vi "Cam1.vi"(1 "error in (no error)":errorcluster) -> (0 "error out":errorcluster caption="error in (no error)")   [LabVIEW 2018]
uses:
  InOut/Reslut.vi
  VsyCam.dll
panel:
  out "当前曝光":dbl
  out "近场图":T1(plugin-control)
  in  "重新连接相机":bool
  out "帧率":dbl
  in  "采集":bool
  in  "数据输出":i32[](listbox)
  out "通信":bool
  out "远场图":T1(plugin-control)
  in  "触发方式":enum8{"软件触发", "上升沿触发", "下降沿触发"}(ring)
  in  "曝光设置 us":i32 min=1 max=2000
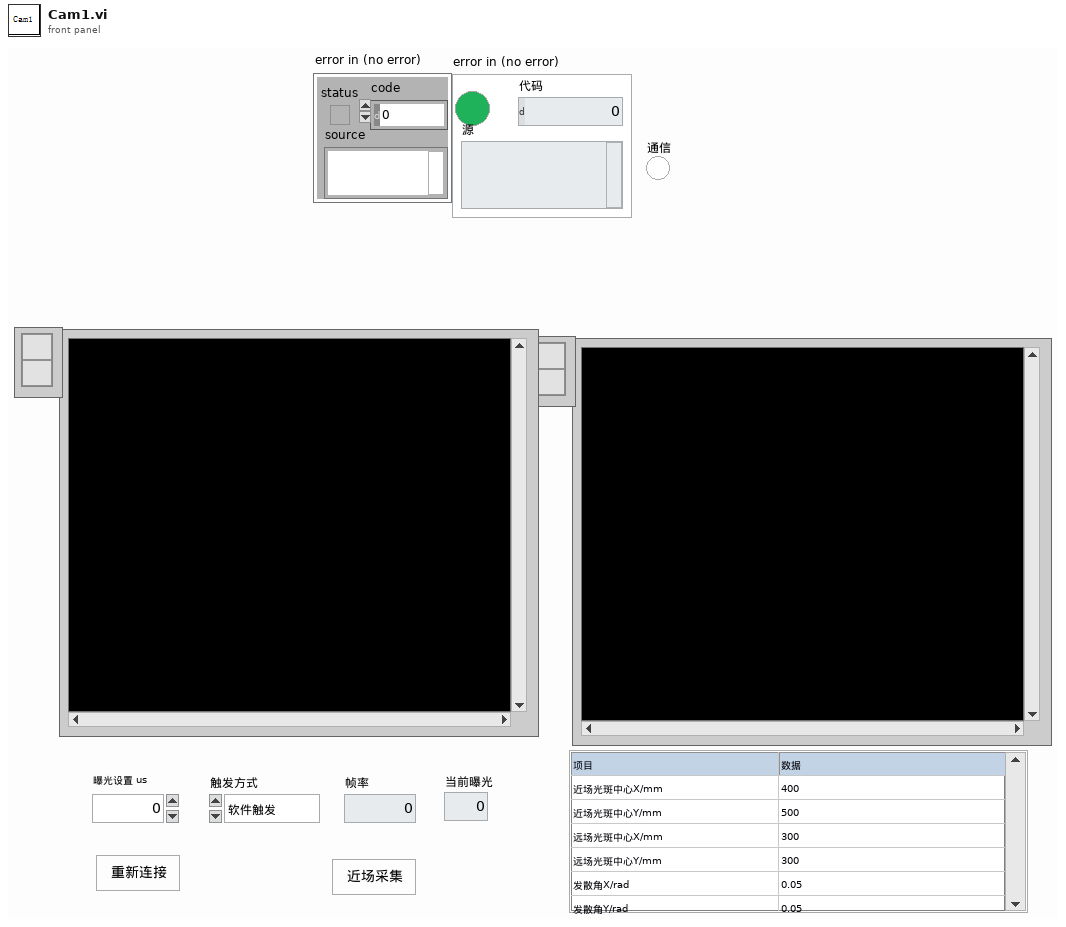
[diagram p1: front panel]
types:
  T1 = typedef "IMAQ Image.ctl" = refnum<image>
  T2 = typedef "Image Type" = u32
  T3 = cluster{"示波器":cluster{"Channel (0:Channel 1)":enum16{"Channel 1", "Channel 2", "Channel 3", "Channel 4"}, "电压范围":dbl, "触发电压":dbl, "时间范围":dbl, " 示波器VISA":refnum<visa-resource-name>, "电压范围 标签":u64, "时间范围 标签":u64}, "光谱仪":cluster{"Channel (0:Channel 1)":enum16{"Channel 1", "Channel 2", "Channel 3", "Channel 4"}, "电压范围":u64, "触发电压":u64, "时间范围":u64}, " 近场相机":cluster{"曝光时间":i32, "模拟增益":i32, "控制套接字":i32, "IP 地址":string, " 采集套接字":i32, "  版本号":i32, "ImageData":T1, "  增益最大":i32, "  增益最小":i32, " 曝光最大":i32, " 曝光最小":i32, " 帧速":i32, " 同步切换":i32, "  曝光缩放":i32}, " 偏振仪":cluster{"电压范围":u64, "触发电压":u64, "时间范围":u64, "波长范围":enum16{"可见光 400-700nm", "近红外 700-1100nm"}}, " 功率计":cluster{"通道":enum16{"Channel 1", "Channel 2"}, "工作波长":u32, "单位":u64, "时间范围":u64, "IP地址":string, "端口":u32}, "能量计":cluster{"通道":enum16{"Channel 1", "Channel 2"}, "工作波长":u32, "单位":u64, "时间范围":u64, "IP地址":string, "端口":u32, "能量计量程":enum16{"200uJ", "20uJ", "2uJ", "200nJ"}}, "电机":cluster{"Channel (0:Channel 1)":enum16{"Channel 1", "Channel 2", "Channel 3", "Channel 4"}, "电压范围":u64, "触发电压":u64, "时间范围":u64}, " 远场相机":cluster{"曝光时间":i32, "模拟增益":i32, "控制套接字":i32, "IP 地址":string, " 采集套接字":i32, "  版本号":i32, "ImageData":T1, "  增益最大":i32, "  增益最小":i32, " 曝光最大":i32, " 曝光最小":i32, " 帧速":i32, " 同步切换":i32, "  曝光缩放":i32}}
  T4 = enum16{"功率测量", "能量测量", "光谱测量", "时间波形", "偏振测量", "近远场"}
  T5 = cluster{"近场图":T1, " 远场图":T1, "发散角X/rad":dbl, "发散角Y/rad":dbl}
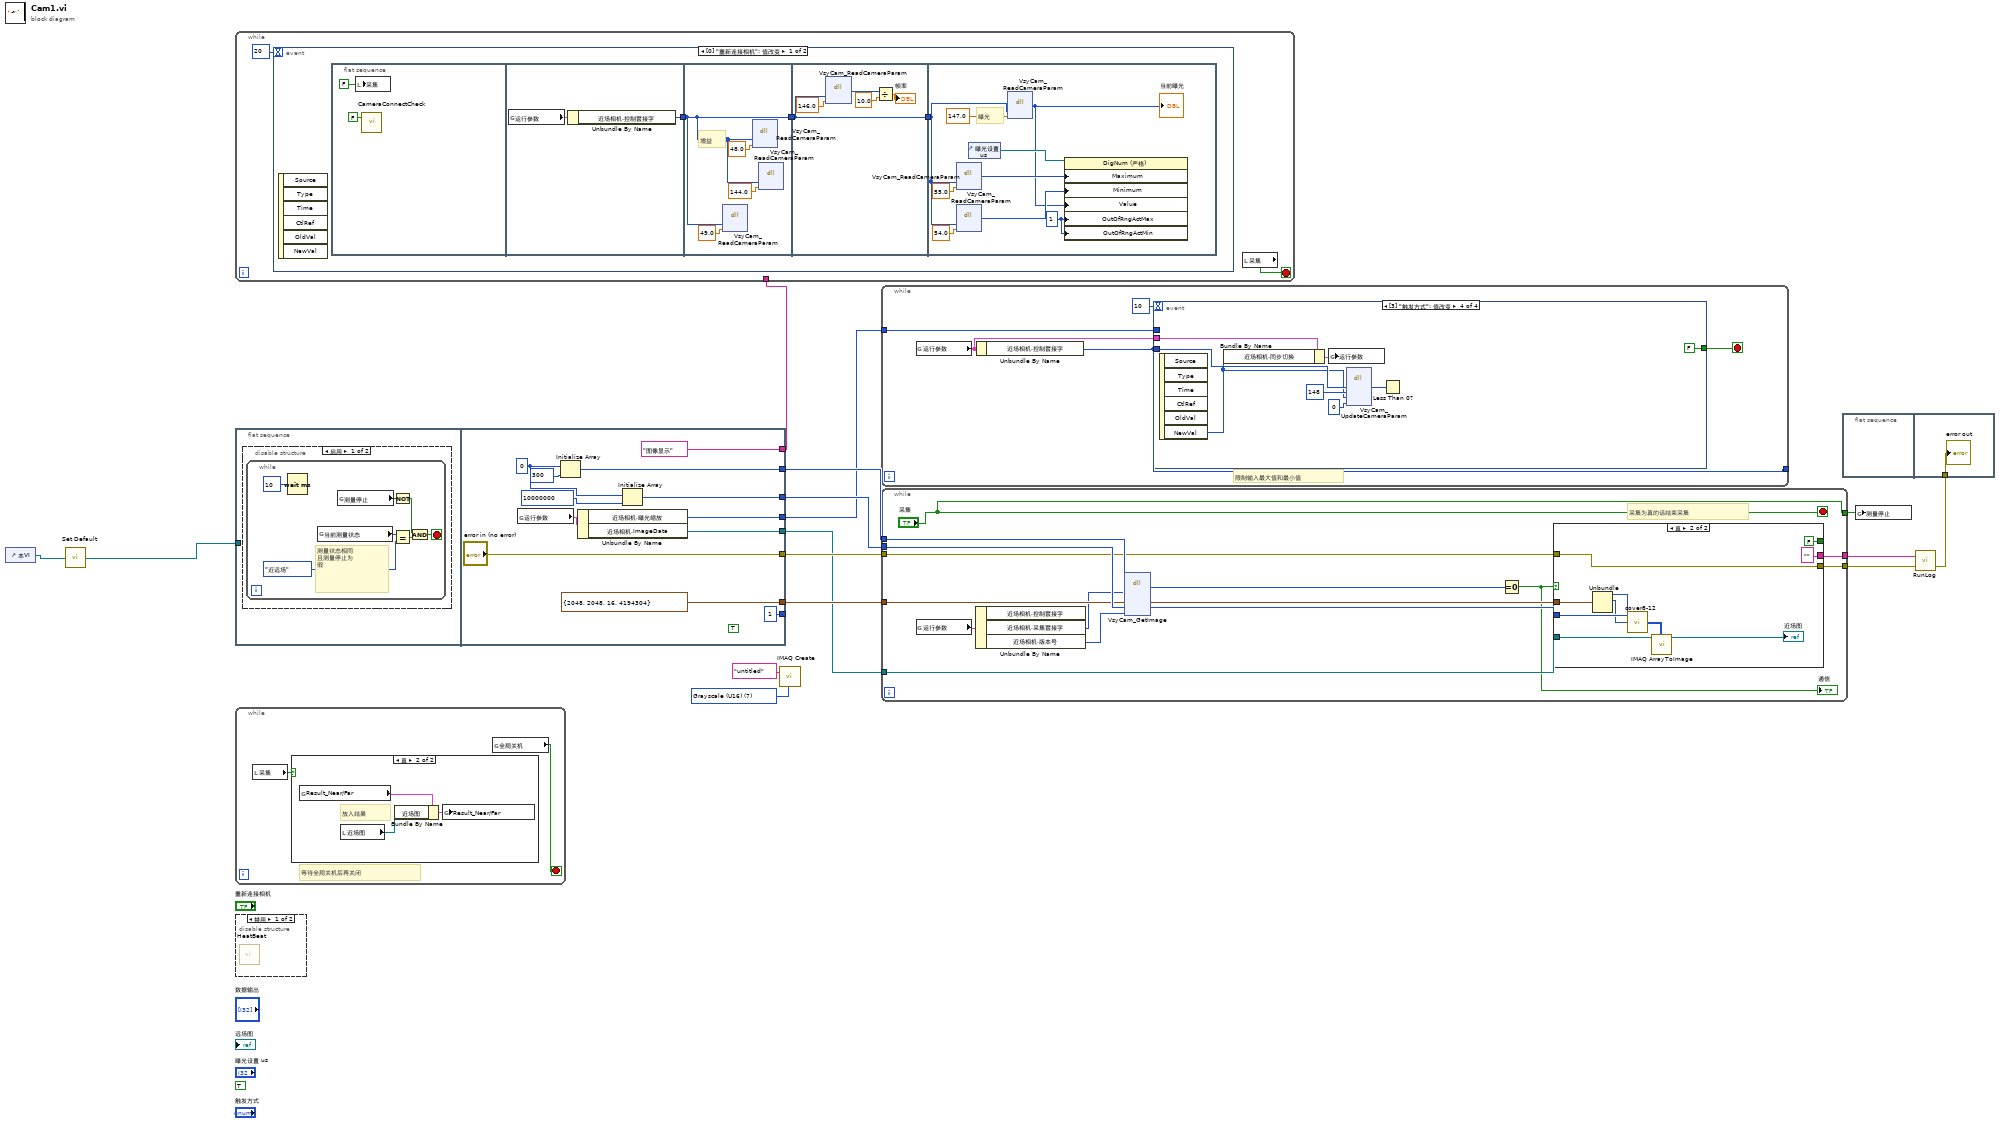
[diagram p0: block diagram]
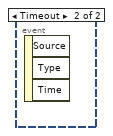
[diagram p3: hidden frame]
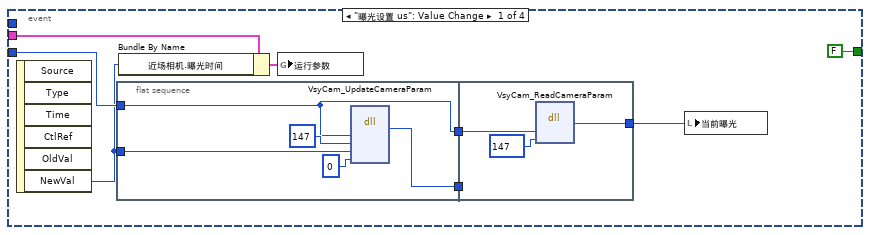
[diagram p6: hidden frame]
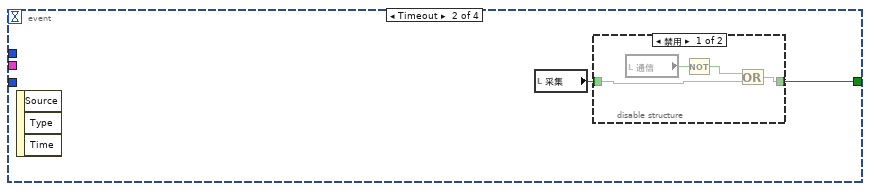
[diagram p7: hidden frame]
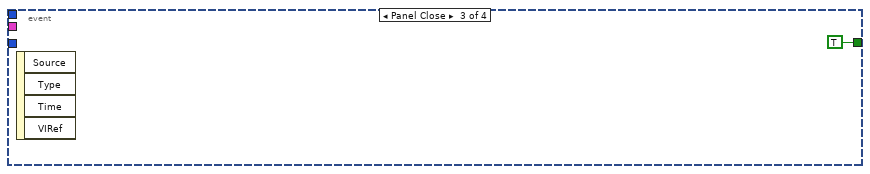
[diagram p9: hidden frame]
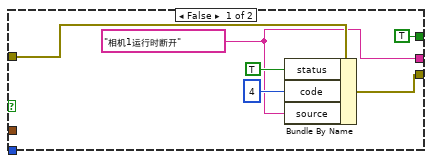
[diagram p10: hidden frame]
diagram:
  w5 = T2 7 items=["Grayscale (U8)", "Grayscale (I16)", "Grayscale (SGL)", "Complex (CSG)", "RGB (U32)", "HSL (U32)", "RGB (U64)", "Grayscale (U16)"] ("Image Type")
  (unwired) TRUE ("Zoom to Fit Mode")
  n1 = control-ref of="本VI"() -> (w4:refnum<vi>)
  n2 = call "Set Default.vi"("VI引用"=w4) -> ("引用输出"=w3:refnum<vi>)
  n3 = while {
    tunnel: w2 -> [_]
    stop <- w17 stop-if-true
    n4 = event shown="[0] \"重新连接相机\": 值改变" {
      selector: _ -> [_ _]
      dyn-events: _ -> [_ _]
      timeout: 20 -> [_ _]
      event "重新连接相机": Value Change {
        n5 = event-data() -> ()  [unwired: 1 in, 6 out]
        n6 = flat-sequence {
          tunnel: [w23] -> w20
          tunnel: w20 -> [w25]
          tunnel: [w25] -> w19
          tunnel: w19 -> [w29]
          tunnel: [w29] -> w18
          tunnel: w18 -> [w37]
          frame #0 {
            n7 = local write "采集"(FALSE ("采集")) -> ()
            n8 = call "CameraConnectCheck.vi"("是否通信检查"=FALSE) -> ()  [unwired: 1 in, 2 out]
          }
          frame #1 {
            n9 = global read "参数.vi" "运行参数"() -> (w24:T3)
            n10 = Unbundle By Name(w24) -> ("近场相机.控制套接字"=w23:i32)
          }
          frame #2 {
            # "增益"
            n11 = dll-call lib="PTH2?abs D做的项目航天测量软件相机\nVsyCam.dll" fn="VsyCam_ReadCameraParam"("sockFd"=w25, "cmd"=49.0) -> ()  [unwired: 6 in, 2 out]
            n12 = dll-call lib="PTH2?abs D做的项目航天测量软件相机\nVsyCam.dll" fn="VsyCam_ReadCameraParam"("sockFd"=w25, "cmd"=48.0) -> ()  [unwired: 6 in, 2 out]
            n13 = dll-call lib="PTH2?abs D做的项目航天测量软件相机\nVsyCam.dll" fn="VsyCam_ReadCameraParam"("sockFd"=w25, "cmd"=144.0) -> ()  [unwired: 6 in, 2 out]
          }
          frame #3 {
            n14 = dll-call lib="PTH2?abs D做的项目航天测量软件相机\nVsyCam.dll" fn="VsyCam_ReadCameraParam"("sockFd"=w29, "cmd"=146.0) -> ("返回类型"=w32:i32)  [unwired: 5 in, 2 out]
            n15 = Divide(x=w32, y=10.0) -> (x/y=→"帧率":dbl)
          }
          frame #4 {
            w38 = u8 1 ("对超出界限的值的响应:最大值")
            # "曝光"
            n16 = dll-call lib="PTH2?abs D做的项目航天测量软件相机\nVsyCam.dll" fn="VsyCam_ReadCameraParam"("sockFd"=w37, "cmd"=55.0) -> ("返回类型"=w36:i32)  [unwired: 5 in, 2 out]
            n17 = dll-call lib="PTH2?abs D做的项目航天测量软件相机\nVsyCam.dll" fn="VsyCam_ReadCameraParam"("sockFd"=w37, "cmd"=54.0) -> ("返回类型"=w35:i32)  [unwired: 5 in, 2 out]
            n18 = control-ref of="曝光设置 us"() -> (w39:refnum<vi>)
            n19 = dll-call lib="PTH2?abs D做的项目航天测量软件相机\nVsyCam.dll" fn="VsyCam_ReadCameraParam"("sockFd"=w37, "cmd"=147.0) -> ("返回类型"=w34:i32)  [unwired: 5 in, 2 out]
            "当前曝光" <- w34
            n20 = property on="属性节点" class="DigNum (严格)"(reference=w39, "Maximum"=w36, "Minimum"=w35, "Value"=w34, "OutOfRngActMax"=w38, "OutOfRngActMin"=w38) -> ()  [unwired: 1 in, 2 out]
          }
        }
      }
      event Timeout {
        n21 = event-data() -> ()  [unwired: 1 in, 3 out]
      }
    }
    n22 = local read "采集"() -> (w17:bool)
  }
  n23 = flat-sequence {
    tunnel: w3 -> [_]
    tunnel: [w58] -> w15
    tunnel: [w57] -> w14
    tunnel: [w52] -> w1
    tunnel: [w56] -> w13
    tunnel: ["error in (no error)"] -> w12
    tunnel: [cluster{i32, i32, i32, i32} {2048, 2048, 16, 4194304} ("簇")] -> w8
    tunnel: ["图像显示" ("名称（未命名）")] -> w2
    tunnel: [1 ("队列最大值（-1，无限）")] -> _
    frame #0 {
      n24 = disable-structure shown="启用" {
        frame Enabled {
          n25 = while {
            stop <- w46 stop-if-true
            # "测量状态相同\n且测量停止为\n假"
            n26 = Wait (ms)(milliseconds to wait=u32 10 ("等待时间（毫秒）")) -> ()  [unwired: 1 out]
            n27 = global read "参数.vi" "当前测量状态"() -> (w44:T4)
            n28 = global read "参数.vi" "测量停止"() -> (w47:bool)
            n29 = Not(x=w47) -> (.not. x?=w48:bool)
            n30 = Equal?(x=w44, y=T4."近远场" ("当前测量状态")) -> (x = y?=w43:bool)
            n31 = And(x=w48, y=w43) -> (x .and. y?=w46:bool)
          }
        }
        frame Disabled {
        }
      }
    }
    frame #1 {
      (unwired) TRUE
      w60 = u8 0
      n32 = global read "参数.vi" "运行参数"() -> (w54:T3)
      n33 = Initialize Array(w60, 300) -> (w58:u8[])
      n34 = Unbundle By Name(w54) -> ("近场相机.曝光缩放"=w56:i32, "近场相机.ImageData"=w52:T1)
      n35 = Initialize Array(w60, 10000000) -> (w57:u8[])
    }
  }
  n36 = while {
    stop <- w63 stop-if-true
    # "等待全局关机后再关闭"
    n37 = local read "采集"() -> (w62:bool)
    n38 = case shown="真" w62 {
      frame False {
      }
      frame True {
        # "放入结果"
        n39 = global read "Reslut.vi" "Result_Near/Far"() -> (w66:T5)
        n40 = local read "近场图"() -> (w64:T1)
        n41 = Bundle By Name(cluster=w66, "近场图"=w64) -> (w65:T5)
        n42 = global write "Reslut.vi" "Result_Near/Far"(w65) -> ()
      }
    }
    n43 = global read "参数.vi" "全局关机"() -> (w63:bool)
  }
  n44 = disable-structure shown="禁用" {
    frame Disabled {
      n45 = call "HeatBeat.vi"() -> ()  [unwired: 12 in]
    }
    frame Enabled {
    }
  }
  n46 = call "IMAQ Create"("Image Name"="untitled", "Image Type"=w5) -> ()  [unwired: 3 in, 2 out]
  n47 = while {
    tunnel: [w68] -> _
    tunnel: w13 -> [w71]
    stop <- w70 stop-if-true
    # "限制输入最大值和最小值"
    n48 = global read "参数.vi" "运行参数"() -> (w67:T3)
    n49 = Unbundle By Name(w67) -> ("近场相机.控制套接字"=w68:i32)
    n50 = event shown="[3] \"触发方式\": 值改变" {
      selector: _ -> [_ _ _ _]
      dyn-events: _ -> [_ _ _ _]
      timeout: 10 -> [_ _ _ _]
      tunnel: w67 -> [w79 _ _ w100]
      tunnel: w68 -> [w78 _ _ w103]
      tunnel: w71 -> [_ _ _ _]
      tunnel: [FALSE w89 TRUE ("近场停止") FALSE] -> w70
      event "曝光设置 us": Value Change {
        n51 = event-data() -> ("NewVal"=w75:i32)  [unwired: 1 in, 5 out]
        n52 = flat-sequence {
          tunnel: w78 -> [w80]
          tunnel: w75 -> [w82]
          tunnel: [w81] -> w74
          tunnel: [w80] -> w73
          tunnel: w74 -> [_]
          tunnel: w73 -> [w87]
          tunnel: [w85] -> w72
          frame #0 {
            n53 = dll-call lib="PTH2?abs D做的项目航天测量软件相机\nVsyCam.dll" fn="VsyCam_UpdateCameraParam"("sockFd"=w80, "command"=147, "value"=w82, "ack"=0) -> ("value"=w81:i32)  [unwired: 7 in, 2 out]
          }
          frame #1 {
            n54 = dll-call lib="PTH2?abs D做的项目航天测量软件相机\nVsyCam.dll" fn="VsyCam_ReadCameraParam"("sockFd"=w87, "cmd"=147) -> ("返回类型"=w85:i32)  [unwired: 5 in, 2 out]
          }
        }
        n55 = Bundle By Name(cluster=w79, "近场相机.曝光时间"=w75) -> (w76:T3)
        n56 = global write "参数.vi" "运行参数"(w76) -> ()
        n57 = local write "当前曝光"(w72) -> ()
      }
      event Timeout {
        n58 = event-data() -> ()  [unwired: 1 in, 3 out]
        n59 = local read "采集"() -> (w88:bool)
        n60 = disable-structure shown="禁用" {
          disable-tunnel: [w92 w94] -> w89
          disable-tunnel: w88 -> [w90 w94]
          frame Disabled {
            n61 = local read "通信"() -> (w91:bool)
            n62 = Not(x=w91) -> (.not. x?=w93:bool)
            n63 = Or(x=w93, y=w90) -> (x .or. y?=w92:bool)
          }
          frame Enabled {
          }
        }
      }
      event Panel Close {
        n64 = event-data() -> ()  [unwired: 1 in, 4 out]
      }
      event "触发方式": Value Change {
        n65 = event-data() -> ("NewVal"=w99:enum8{"软件触发", "上升沿触发", "下降沿触发"})  [unwired: 1 in, 5 out]
        n66 = Bundle By Name(cluster=w100, "近场相机.同步切换"=w99) -> (w96:T3)
        n67 = global write "参数.vi" "运行参数"(w96) -> ()
        n68 = dll-call lib="PTH2?abs D做的项目航天测量软件相机\nVsyCam.dll" fn="VsyCam_UpdateCameraParam"("sockFd"=w103, "command"=148, "value"=w99, "ack"=0) -> ("sockFd"=w98:i32)  [unwired: 7 in, 2 out]
        n69 = Less Than 0?(x=w98) -> ()  [unwired: 1 out]
      }
    }
  }
  n70 = while {
    tunnel: w15 -> [w118]
    tunnel: w14 -> [w116]
    tunnel: w1 -> [w112]
    tunnel: w8 -> [w115]
    tunnel: w12 -> [w111]
    tunnel: [w110] -> w11
    tunnel: [w109] -> w10
    tunnel: ["采集"] -> w7
    stop <- "采集" stop-if-true
    # "采集为真的话结束采集"
    n71 = global read "参数.vi" "运行参数"() -> (w104:T3)
    n72 = Unbundle By Name(w104) -> ("近场相机.采集套接字"=w106:i32, "近场相机.版本号"=w105:i32)  [unwired: 1 out]
    n73 = dll-call lib="PTH2?abs D做的项目航天测量软件相机\nVsyCam.dll" fn="VsyCam_GetImage" label="VsyCam_GetImageVsyCam_GetImage"("sockFd"=w106, "Header"=w118, "ImgInfo"=w115, "Data"=w116, "version"=w105) -> ("返回类型"=w117:i32, "ImgInfo"=w114:cluster{i32, i32, i32, i32}, "Data"=w113:u8[])  [unwired: 6 in, 2 out]
    n74 = Equal To 0?(x=w117) -> (x = 0?=w108:bool)
    "通信" <- w108
    n75 = case shown="真" w108 {
      tunnel: w114 -> [_ w134]
      tunnel: w113 -> [_ w133]
      tunnel: w112 -> [_ w130]
      tunnel: w111 -> [w124 w127]
      tunnel: [w121 w127] -> w110
      tunnel: [TRUE FALSE] -> _
      tunnel: [w119 "" ("source")] -> w109
      frame False {
        w119 = "相机1运行时断开" ("source")
        n76 = Bundle By Name(cluster=w124, "status"=TRUE, "code"=4, "source"=w119) -> (w121:errorcluster)
      }
      frame True {
        n77 = Unbundle(w134) -> (w132:i32, w131:i32)  [unwired: 2 out]
        n78 = call "cover8-12.vi"("H"=w132, "W"=w131, "Image Data"=w133) -> ("PIC Out"=w129:u16[][])
        n79 = call "IMAQ ArrayToImage"("Image Pixels (U16)"=w129, "Image"=w130) -> ("Image Out"=→"近场图":T1)  [unwired: 8 in, 1 out]
      }
    }
  }
  n80 = flat-sequence {
    tunnel: w9 -> [w135]
    frame #0 {
    }
    frame #1 {
      "error out" <- w135
    }
  }
  n81 = global write "参数.vi" "测量停止"(w7) -> ()
  n82 = call "RunLog.vi"("error in"=w11, "Message"=w10) -> ("error out"=w9:errorcluster)  [unwired: 1 in]
